vi "MSScript_Format_AuxScan.vi"(9 "ValueArray":string[](array[string]), 10 "TagArray":string[](array[string]), 11 "MSScript in":refnum<class "MSScript.lvclass">) -> (0 "ValueErrorArray":bool[](array[boolean]), 1 "TagErrorArray":bool[](array[boolean]), 2 "ParamErrorArray":bool[](array[boolean]), 3 "Data":variant, 4 "#ofParamError":bool)   [LabVIEW 2018, in "MSScript.lvclass"]
uses:
  MSScript.lvclass
  Ctl/MSEditorParam auxScan.ctl
  MSScript_Transform_UInt.vi
  MSScript_Transform_Extended.vi
  MSScript_Transform_EXTArray.vi
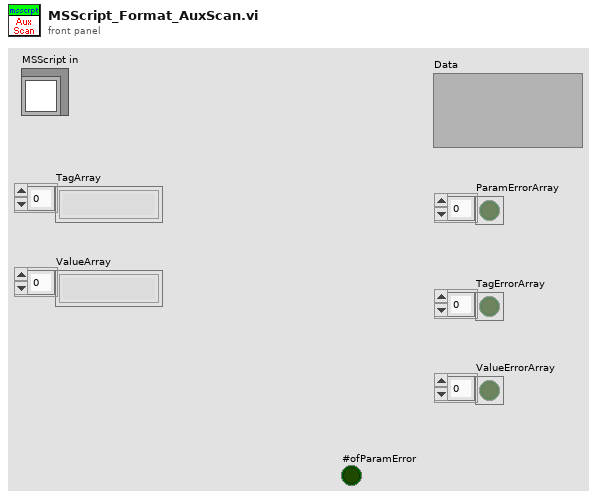
[diagram p1: front panel]
types:
  T1 = typedef "MSEditorParam auxScan.ctl" = cluster{"auxWfmType":u32, "auxStart":u32, "iauxCyc":ext, "auxCyc":ext[], "beta":ext[], "betaScale":ext, "auxAmp":ext[], "auxPulse1":ext[], "auxPulse2":ext[], "auxPulseAmp":ext[], "time":ext}
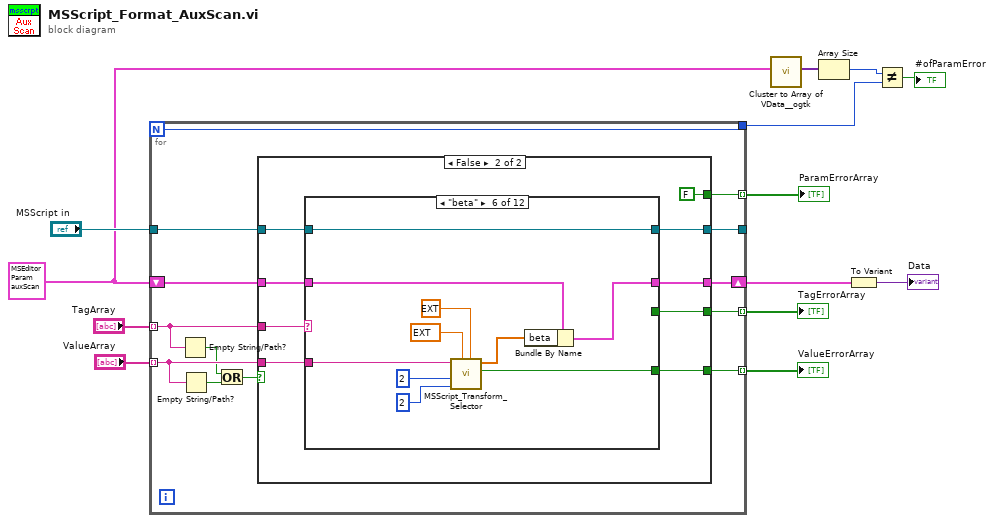
[diagram p0: block diagram]
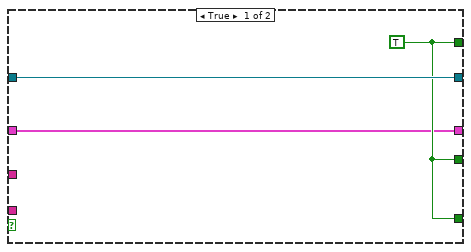
[diagram p2: hidden frame]
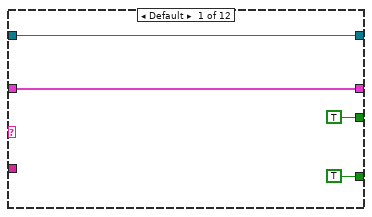
[diagram p3: hidden frame]
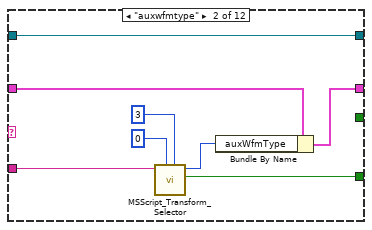
[diagram p4: hidden frame]
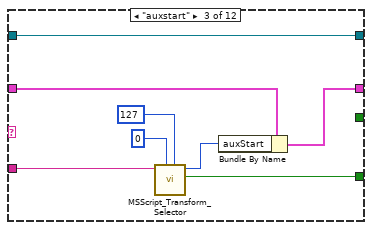
[diagram p5: hidden frame]
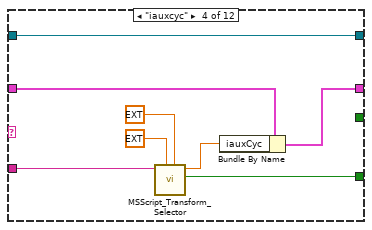
[diagram p6: hidden frame]
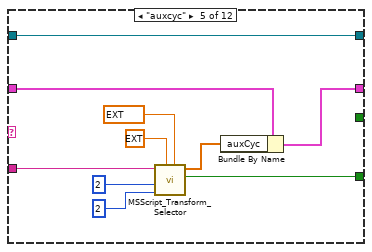
[diagram p7: hidden frame]
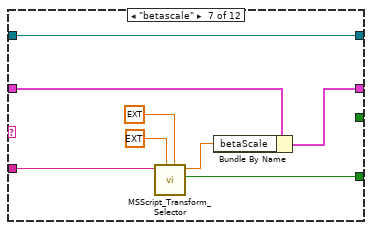
[diagram p8: hidden frame]
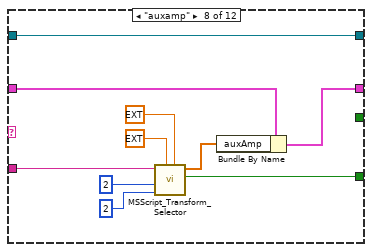
[diagram p9: hidden frame]
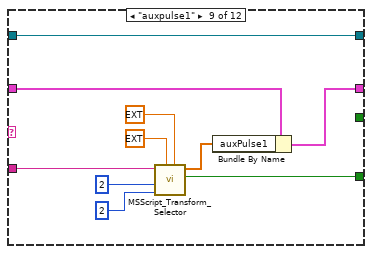
[diagram p10: hidden frame]
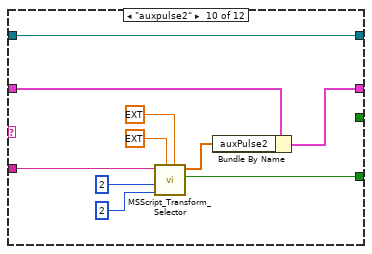
[diagram p11: hidden frame]
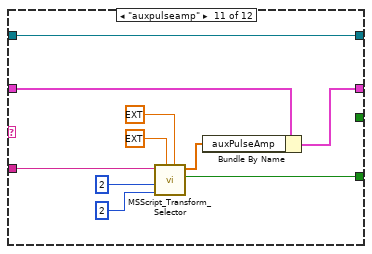
[diagram p12: hidden frame]
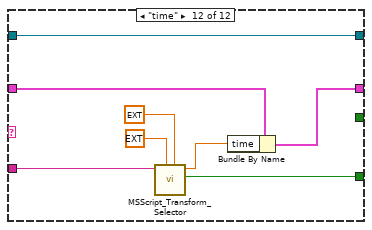
[diagram p13: hidden frame]
diagram:
  w3 = T1 {"auxWfmType"=0, "auxStart"=0, "iauxCyc"=0.0, "auxCyc"=[1.0, 1.0], "beta"=[0.1, 0.5], "betaScale"=1.0, "auxAmp"=[1.0, 1.0], "auxPulse1"=[0.0, 0.5], "auxPulse2"=[0.5, 1.0], "auxPulseAmp"=[1.0, -1.0], "time"=1.0} ("ParamValueType")
  n1 = for {
    N -> [w14]
    tunnel: "TagArray" -> [w22] mode=indexing
    tunnel: "ValueArray" -> [w21] mode=indexing
    tunnel: [w26] -> w11 mode=indexing
    tunnel: "MSScript in" -> [w25]
    tunnel: [w24] -> w10 mode=indexing
    tunnel: [w23] -> _
    tunnel: [w17] -> w9 mode=indexing
    shift-right: [w15] -> w7
    shift-left: w3 -> [w16]
    tunnel: [w14] -> w2
    n2 = Empty String/Path?(string/path=w22) -> (empty?=w19:bool)
    n3 = Empty String/Path?(string/path=w21) -> (empty?=w20:bool)
    n4 = Or(x=w19, y=w20) -> (x .or. y?=w18:bool)
    n5 = case shown="False" w18 {
      tunnel: [w28 w32] -> w26
      tunnel: w25 -> [w29 w37]
      tunnel: [w28 w30] -> w24
      tunnel: [w29 w31] -> w23
      tunnel: w22 -> [_ w35]
      tunnel: w21 -> [_ w34]
      tunnel: [w28 FALSE] -> w17
      tunnel: w16 -> [w27 w36]
      tunnel: [w27 w33] -> w15
      frame True {
        w28 = TRUE
      }
      frame False {
        n6 = case shown="\"beta\"" w35 {
          tunnel: [TRUE _ _ _ _ _ _ _ _ _ _ _] -> w32
          tunnel: w37 -> [w40 w48 w56 w64 w74 w84 w92 w102 w112 w122 w132 w140]
          tunnel: w34 -> [_ w49 w57 w65 w75 w85 w93 w103 w113 w123 w133 w141]
          tunnel: [TRUE ("Value Error?") w50 w58 w66 w76 w86 w94 w104 w114 w124 w134 w142] -> w30
          tunnel: [w40 w48 w56 w64 w74 w84 w92 w102 w112 w122 w132 w140] -> w31
          tunnel: w36 -> [w39 w46 w54 w62 w72 w82 w90 w100 w110 w120 w130 w138]
          tunnel: [w39 w45 w53 w61 w71 w81 w89 w99 w109 w119 w129 w137] -> w33
          frame Default {
          }
          frame "auxwfmtype" {
            n7 = call-poly "MSScript_Transform_Selector.vi"("upper limit"=u64 3, "lower limit"=u64 0, "string in"=w49) -> ("Value Error?"=w50:bool, "Value Output"=w47:u64)  [unwired: 6 in, 1 out]
            n8 = Bundle By Name(cluster=w46, "auxWfmType"=w47) -> (w45:T1)
          }
          frame "auxstart" {
            n9 = call-poly "MSScript_Transform_Selector.vi"("upper limit"=u64 127, "lower limit"=u64 0, "string in"=w57) -> ("Value Error?"=w58:bool, "Value Output"=w55:u64)  [unwired: 6 in, 1 out]
            n10 = Bundle By Name(cluster=w54, "auxStart"=w55) -> (w53:T1)
          }
          frame "iauxcyc" {
            n11 = call-poly "MSScript_Transform_Selector.vi"("upper limit (Inf)"=ext 1.0 ("upper limit"), "lower limit (-Inf)"=ext 0.0 ("lower limit"), "Check_Str"=w65) -> ("Value Error?"=w66:bool, "Value Output"=w63:ext)  [unwired: 6 in, 1 out]
            n12 = Bundle By Name(cluster=w62, "iauxCyc"=w63) -> (w61:T1)
          }
          frame "auxcyc" {
            n13 = call-poly "MSScript_Transform_Selector.vi"("upper limit (Inf)"=ext 99999.0 ("upper limit"), "lower limit (-Inf)"=ext 0.0 ("lower limit"), "MinSize"=u8 2, "MaxSize"=u8 2, "check_str"=w75) -> ("Value Error?"=w76:bool, "Value Output"=w73:ext[])  [unwired: 4 in, 1 out]
            n14 = Bundle By Name(cluster=w72, "auxCyc"=w73) -> (w71:T1)
          }
          frame "beta" {
            n15 = call-poly "MSScript_Transform_Selector.vi"("upper limit (Inf)"=ext 1.0 ("upper limit"), "lower limit (-Inf)"=ext 0.01 ("lower limit"), "MinSize"=u8 2, "MaxSize"=u8 2, "check_str"=w85) -> ("Value Error?"=w86:bool, "Value Output"=w83:ext[])  [unwired: 4 in, 1 out]
            n16 = Bundle By Name(cluster=w82, "beta"=w83) -> (w81:T1)
          }
          frame "betascale" {
            n17 = call-poly "MSScript_Transform_Selector.vi"("upper limit (Inf)"=ext 10.0 ("upper limit"), "lower limit (-Inf)"=ext 0.0 ("lower limit"), "Check_Str"=w93) -> ("Value Error?"=w94:bool, "Value Output"=w91:ext)  [unwired: 6 in, 1 out]
            n18 = Bundle By Name(cluster=w90, "betaScale"=w91) -> (w89:T1)
          }
          frame "auxamp" {
            n19 = call-poly "MSScript_Transform_Selector.vi"("upper limit (Inf)"=ext 1.0 ("upper limit"), "lower limit (-Inf)"=ext 0.0 ("lower limit"), "MinSize"=u8 2, "MaxSize"=u8 2, "check_str"=w103) -> ("Value Error?"=w104:bool, "Value Output"=w101:ext[])  [unwired: 4 in, 1 out]
            n20 = Bundle By Name(cluster=w100, "auxAmp"=w101) -> (w99:T1)
          }
          frame "auxpulse1" {
            n21 = call-poly "MSScript_Transform_Selector.vi"("upper limit (Inf)"=ext 1.0 ("upper limit"), "lower limit (-Inf)"=ext 0.0 ("lower limit"), "MinSize"=u8 2 ("MaxSize"), "MaxSize"=u8 2, "check_str"=w113) -> ("Value Error?"=w114:bool, "Value Output"=w111:ext[])  [unwired: 4 in, 1 out]
            n22 = Bundle By Name(cluster=w110, "auxPulse1"=w111) -> (w109:T1)
          }
          frame "auxpulse2" {
            n23 = call-poly "MSScript_Transform_Selector.vi"("upper limit (Inf)"=ext 1.0 ("upper limit"), "lower limit (-Inf)"=ext 0.0 ("lower limit"), "MinSize"=u8 2 ("MaxSize"), "MaxSize"=u8 2, "check_str"=w123) -> ("Value Error?"=w124:bool, "Value Output"=w121:ext[])  [unwired: 4 in, 1 out]
            n24 = Bundle By Name(cluster=w120, "auxPulse2"=w121) -> (w119:T1)
          }
          frame "auxpulseamp" {
            n25 = call-poly "MSScript_Transform_Selector.vi"("upper limit (Inf)"=ext 1.0 ("upper limit"), "lower limit (-Inf)"=ext -1.0 ("lower limit"), "MinSize"=u8 2 ("MaxSize"), "MaxSize"=u8 2, "check_str"=w133) -> ("Value Error?"=w134:bool, "Value Output"=w131:ext[])  [unwired: 4 in, 1 out]
            n26 = Bundle By Name(cluster=w130, "auxPulseAmp"=w131) -> (w129:T1)
          }
          frame "time" {
            n27 = call-poly "MSScript_Transform_Selector.vi"("upper limit (Inf)"=ext 60.0 ("upper limit"), "lower limit (-Inf)"=ext 0.0 ("lower limit"), "Check_Str"=w141) -> ("Value Error?"=w142:bool, "Value Output"=w139:ext)  [unwired: 6 in, 1 out]
            n28 = Bundle By Name(cluster=w138, "time"=w139) -> (w137:T1)
          }
        }
      }
    }
  }
  "TagErrorArray" <- w11
  "ValueErrorArray" <- w10
  "ParamErrorArray" <- w9
  n29 = call <userlib>:"Cluster to Array of VData__ogtk.vi"("Cluster"=w3) -> ("Array of VData"=w6:variant[])  [unwired: 9 in, 1 out]
  n30 = Array Size(array=w6) -> (size(s)=w5:i32)
  n31 = To Variant(anything=w7) -> (Variant=→"Data":variant)
  n32 = Not Equal?(x=w5, y=w2) -> (x != y?=→"#ofParamError":bool)
